vi "Update DIO Registers.vi"(8 "error in (no error)":errorcluster, 9 "Output?":bool[](array[boolean]), 10 "Direction":bool[](array[boolean]), 11 "Data":T1) -> (0 "error out":errorcluster)   [LabVIEW 2017, in "Test Bench.lvlib"]
uses:
  Test Bench.lvlib
  Scan Engine Variables.ctl
  <instrlib>/_niInstr/FIFO Register Bus/v1/Host/niInstr FIFO Register Bus v1 Host.lvclass
  C:/Program Files (x86)/National Instruments/LabVIEW 2017/instr.lib/_niInstr/Instruction Framework/v1/Host/Instruction Target/niInstr Instruction Target v1 Host.lvclass
  <instrlib>/_niInstr/Instruction Framework/v1/Host/Instruction Framework Context/niInstr Instruction Framework Context v1 Host.lvclass
  <instrlib>/_niInstr/Instruction Framework/v1/Host/Instruction Target/niInstr Instruction Target v1 Host.lvclass
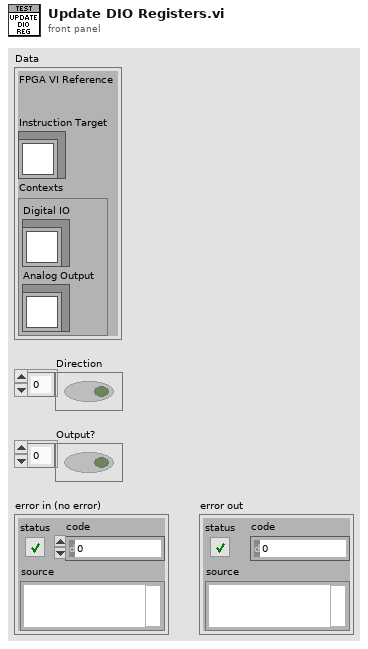
[diagram p1: front panel]
types:
  T1 = typedef "Test Bench.lvlib/Scan Engine Variables.ctl" = cluster{"FPGA VI Reference":refnum<k20>, "Instruction Target":refnum<class "niInstr FIFO Register Bus v1 Host.lvclass">, "Contexts":cluster{"Digital IO":refnum<class "niInstr Instruction Framework Context v1 Host.lvclass">, "Analog Output":refnum<class "niInstr Instruction Framework Context v1 Host.lvclass">}}
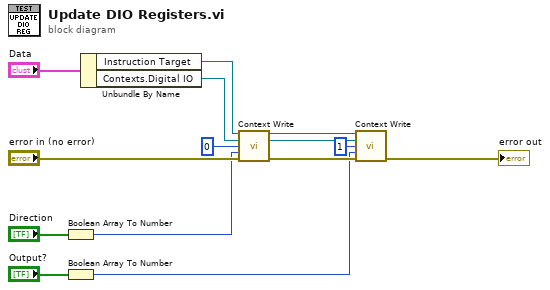
[diagram p0: block diagram]
diagram:
  n1 = Boolean Array To Number(Boolean array="Direction") -> (number=w2:u64)
  n2 = Boolean Array To Number(Boolean array="Output?") -> (number=w4:u64)
  n3 = Unbundle By Name("Data") -> ("Instruction Target"=w14:refnum<class "niInstr FIFO Register Bus v1 Host.lvclass">, "Contexts.Digital IO"=w11:refnum<class "niInstr Instruction Framework Context v1 Host.lvclass">)
  n4 = call <instrlib>:"Context Write.vi"("instruction target in"=w14, "context in"=w11, "address"=u64 0, "data"=w2, "error in"="error in (no error)") -> ("instruction target out"=w13:refnum<class "niInstr FIFO Register Bus v1 Host.lvclass">, "context out"=w12:refnum<class "niInstr Instruction Framework Context v1 Host.lvclass">, "error out"=w8:errorcluster)  [unwired: 8 in]
  n5 = call <instrlib>:"Context Write.vi"("instruction target in"=w13, "context in"=w12, "address"=u64 1, "data"=w4, "error in"=w8) -> ("error out"=→"error out":errorcluster)  [unwired: 8 in, 2 out]
